vi "GetWAVData.vi"(8 "error in (no error)":errorcluster, 10 "WAV file path":path, 11 "Channel":string) -> (0 "error out":errorcluster, 3 "DataSet":T1)   [LabVIEW 2017, in "EmsaTestPanel.lvlib"]
uses:
  <vilib>/addons/InsightCM/Devices/Shared/Emsa/EmsaTestPanel/EmsaTestPanel.lvlib
  <vilib>/addons/InsightCM/MessageBus/Base/controls/DataSetByteData.ctl
  <vilib>/addons/InsightCM/MessageBus/Base/controls/KeyValuePair.ctl
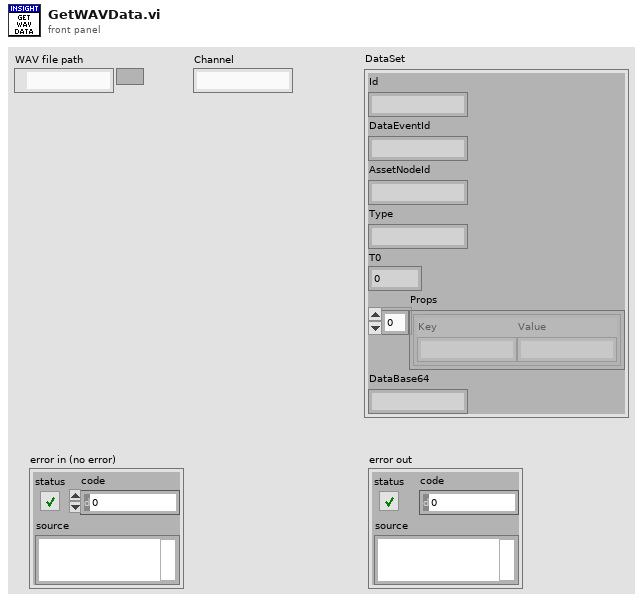
[diagram p1: front panel]
types:
  T1 = typedef "DataSetByteData.ctl" = cluster{"Id":string, "DataEventId":string, "AssetNodeId":string, "Type":string, "T0":i64, "Props":T2[], "DataBase64":string}
  T2 = typedef "KeyValuePair.ctl" = cluster{"Key":string, "Value":string}
  T3 = enum16{"big-endian, network order", "native, host order", "little-endian"}
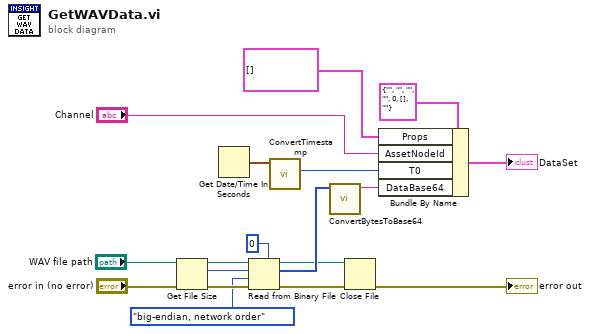
[diagram p0: block diagram]
diagram:
  n1 = Get File Size(file="WAV file path", error in="error in (no error)") -> (refnum out=w8:refnum<file>, size (in bytes)=w5:i64, 0:w6:errorcluster)
  n2 = Get Date/Time In Seconds() -> (seconds since 1Jan1904=w13:timestamp)
  n3 = Read from Binary File(5:u8 0 ("Numeric"), 8:w6, 9:T3."big-endian, network order" ("byte order (0:big-endian, network order)"), 10:w5, 11:w8) -> (0:w3:errorcluster, 2:w16:u8[], 3:w2:refnum<file>)  [unwired: 1 in, 1 out]
  n4 = call <vilib>:"ConvertTimestamp.vi"("Time Stamp"=w13) -> ("Timestamp out"=w12:i64)  [unwired: 10 in]
  n5 = call <vilib>:"ConvertBytesToBase64.vi"("U8 array"=w16) -> ("base64 encoded"=w11:string)  [unwired: 10 in]
  n6 = Close File(refnum=w2, error in=w3) -> (error out=→"error out":errorcluster)  [unwired: 1 out]
  n7 = Bundle By Name(cluster=T1 {"Id"="", "DataEventId"="", "AssetNodeId"="", "Type"="", "T0"=0, "Props"=[], "DataBase64"=""} ("DataSet"), "Props"=T2[] [] ("key value pairs"), "AssetNodeId"="Channel", "T0"=w12, "DataBase64"=w11) -> (→"DataSet":T1)
